vi "get configuration.vi"(8 "Serial Port":refnum<visa-resource-name>) -> (3 "zones":T1, 4 "Serial Port":refnum<visa-resource-name>, 5 "Detectors":T2)   [LabVIEW 2012]
uses:
  detector.ctl
  zones.ctl
panel:
  out "Det B zone":bool
  out "Det A zone":bool
  out "Inj B zone":bool
  out "Inj A zone":bool
  out "Det B":string
  out "Det A":string
  out "response":string
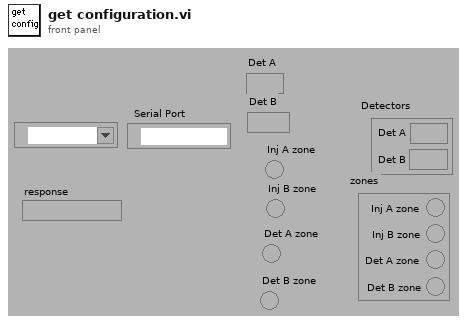
[diagram p1: front panel]
types:
  T1 = typedef "zones.ctl" = cluster{"Inj A zone":bool, "Det A zone":bool, "Inj B zone":bool, "Det B zone":bool}
  T2 = typedef "detector.ctl" = cluster{"Det A":string, "Det B":string}
  T3 = cluster{"[0]":bool, "[1]":bool, "[2]":bool, "[3]":bool}
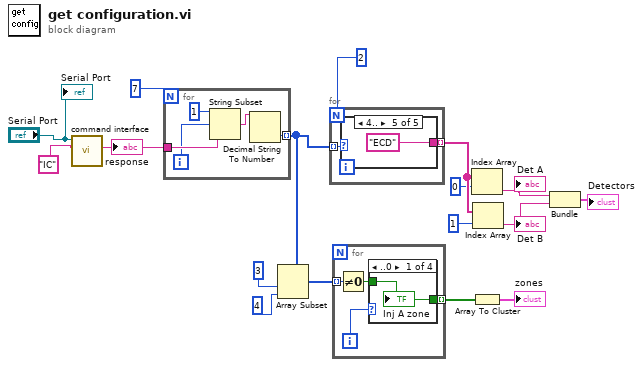
[diagram p0: block diagram]
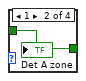
[diagram p2: hidden frame]
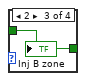
[diagram p3: hidden frame]
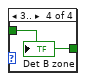
[diagram p4: hidden frame]
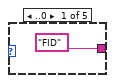
[diagram p5: hidden frame]
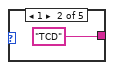
[diagram p6: hidden frame]
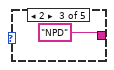
[diagram p7: hidden frame]
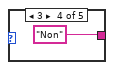
[diagram p8: hidden frame]
diagram:
  n1 = call "command interface.vi"("command"="IC", "Serial Port"="Serial Port") -> ("response"=w16:string)  [unwired: 5 in, 3 out]
  "response" <- w16
  n2 = for {
    N: 7 -> [_]
    tunnel: w16 -> [w20]
    tunnel: [w22] -> w10 mode=indexing
    i -> [w19]
    n3 = String Subset(string=w20, offset (0)=w19, length (rest)=1) -> (substring=w18:string)
    n4 = Decimal String To Number(string=w18) -> (number=w22:i32)  [unwired: 2 in, 1 out]
  }
  n5 = Array Subset(array=w10, index=3, length=4) -> (w7:i32[])
  n6 = for {
    N: 2 -> [_]
    tunnel: w10 -> [w24] mode=indexing
    tunnel: [w23] -> w13 mode=indexing
    n7 = case shown="4.." w24 {
      tunnel: ["FID" "TCD" "NPD" "Non" "ECD"] -> w23
      frame ..0 {
      }
      frame 1 {
      }
      frame 2 {
      }
      frame 3 {
      }
      frame 4.. {
      }
    }
  }
  n8 = for {
    tunnel: w7 -> [w33] mode=indexing
    tunnel: [w30] -> w1 mode=indexing
    i -> [w32]
    n9 = Not Equal To 0?(x=w33) -> (x != 0?=w31:bool)
    n10 = case shown="..0" w32 {
      tunnel: w31 -> [w34 w35 w36 w37]
      tunnel: [w34 w35 w36 w37] -> w30
      frame ..0 {
        "Inj A zone" <- w34
      }
      frame 1 {
        "Det A zone" <- w35
      }
      frame 2 {
        "Inj B zone" <- w36
      }
      frame 3.. {
        "Det B zone" <- w37
      }
    }
  }
  n11 = Index Array(array=w13, index=0) -> (element=w4:string)
  "Det A" <- w4
  n12 = Array To Cluster(array=w1) -> (cluster=→"zones":T3)
  n13 = Index Array(array=w13, index=1) -> (element=w5:string)
  "Det B" <- w5
  n14 = Bundle(w4, w5) -> (→"Detectors":cluster{string, string})  [unwired: 1 in]
  "Serial Port" <- "Serial Port"
